vi "Revision Query Core.vi"(8 "error in (no error)":errorcluster, 11 "LS218 in":refnum<class "LS218.lvclass">) -> (0 "error out":errorcluster, 1 "Firmware Revision":string, 2 "Driver Revision":string, 3 "LS218 out":refnum<class "LS218.lvclass">)   [LabVIEW 2013, in "LS218.lvlib" / "LS218.lvclass"]
uses:
  LS218.lvclass
  CSPP_Core/Actors/CS++DeviceActor/CS++DeviceActor.lvclass
  LS218.lvclass/LS218.ctl
  <instrlib>/Lake Shore Cryotronics 218/Lake Shore Cryotronics 218.lvlib
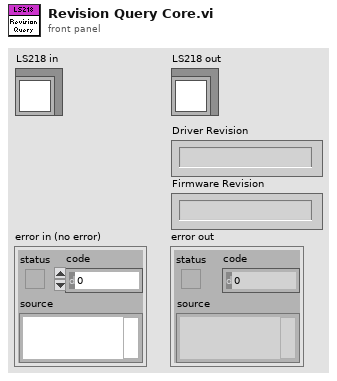
[diagram p1: front panel]
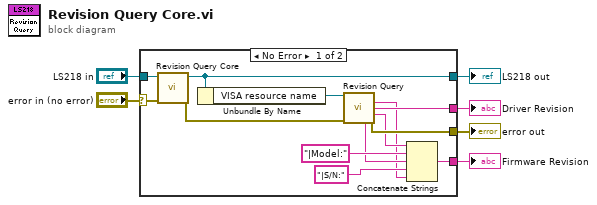
[diagram p0: block diagram]
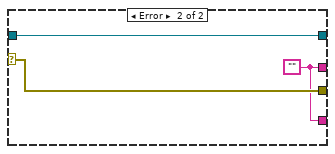
[diagram p2: hidden frame]
diagram:
  n1 = case shown="No Error" "error in (no error)" {
    selector: "error in (no error)" -> [w7 w21]
    tunnel: "LS218 in" -> [w19 w22]
    tunnel: [w18 w22] -> w5
    tunnel: [w15 w21] -> w4
    tunnel: [w14 w20] -> w3
    tunnel: [w8 w20] -> w2
    frame No Error {
      n2 = call-parent "Revision Query Core.vi"("error in (no error)"=w7, "CS++DeviceActor in"=w19) -> ("error out"=w16:errorcluster, "CS++DeviceActor out"=w18:refnum<class "LS218.lvclass">)  [unwired: 6 in, 2 out]
      n3 = Unbundle By Name(w18) -> ("VISA resource name"=w17:refnum<visa-resource-name>)
      n4 = call <instrlib>:"Revision Query.vi"("VISA resource name"=w17, "error in (no error)"=w16) -> ("Instr Serial Number"=w9:string, "Instr Driver Revision"=w14:string, "Instr Firmware Revision"=w13:string, "Instr Model Number"=w11:string, "error out"=w15:errorcluster)  [unwired: 8 in, 1 out]
      n5 = Concatenate Strings(w13, "|Model:" ("string"), w11, "|S/N:" ("string"), w9) -> (w8:string)
    }
    frame Error {
      w20 = ""
    }
  }
  "error out" <- w4
  "LS218 out" <- w5
  "Driver Revision" <- w3
  "Firmware Revision" <- w2
